vi "Convert register values.vi"(10 "Register strings":string[](array[string]), 11 "Register clusters":T1[](array[typedef])) -> (2 "Register clusters out":T1[](array[typedef]), 3 "Register strings out":string[](array[string]))   [LabVIEW 2020, in "PIC-Device.lvclass"]
uses:
  PIC-Device.lvclass
  Controls/Register to Write.ctl
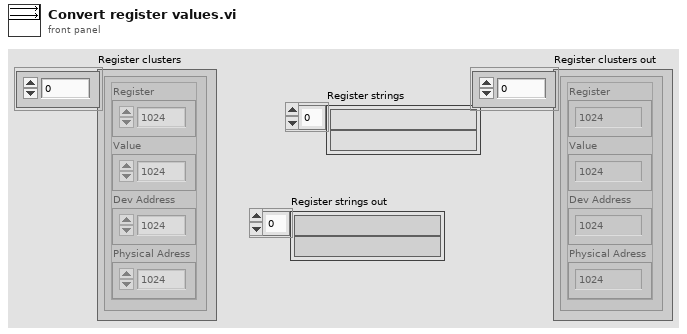
[diagram p1: front panel]
types:
  T1 = typedef "PIC-Device.lvclass/Register to Write.ctl" = cluster{"Register":u32, "Value":u32, "Dev Address":u32, "Physical Adress":u32}
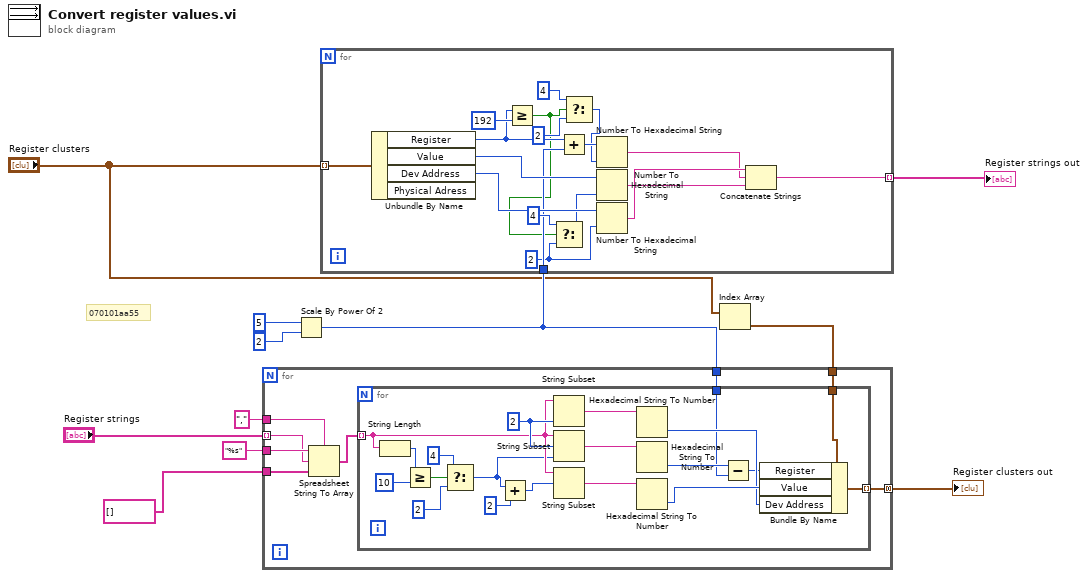
[diagram p0: block diagram]
diagram:
  # "070101aa55"
  n1 = Scale By Power Of 2(n=u32 5, x=u32 2) -> (x*2^n=w9:u32)
  n2 = for {
    tunnel: [w24] -> w7 mode=indexing
    tunnel: "Register clusters" -> [w23] mode=indexing
    tunnel: w9 -> [w15]
    w13 = i16 2 ("width (-)")
    n3 = Unbundle By Name(w23) -> ("Register"=w20:u32, "Value"=w22:u32, "Dev Address"=w28:u32)  [unwired: 1 out]
    n4 = Greater Or Equal?(x=w20, y=u32 192) -> (x >= y?=w12:bool)
    n5 = Select(t=i16 4 ("width (-)"), s=w12, f=w13) -> (s? t:f=w14:i16)
    n6 = Add(x=w20, y=w15) -> (x+y=w29:u32)
    n7 = Select(t=i16 4 ("width (-)"), s=w12, f=i16 2 ("width (-)")) -> (s? t:f=w17:i16)
    n8 = Number To Hexadecimal String(1:w17, 2:w29) -> (0:w26:string)
    n9 = Number To Hexadecimal String(1:w14, 2:w22) -> (0:w25:string)
    n10 = Number To Hexadecimal String(1:w13, 2:w28) -> (0:w27:string)
    n11 = Concatenate Strings(w27, w26, w25) -> (w24:string)
  }
  "Register strings out" <- w7
  n12 = Index Array(array="Register clusters") -> (element=w4:T1)  [unwired: 1 in]
  n13 = for {
    tunnel: "Register strings" -> [w31] mode=indexing
    tunnel: w9 -> [w35]
    tunnel: w4 -> [w37]
    tunnel: [w36] -> w6 mode=concatenating
    tunnel: string[] [] -> [w34]
    tunnel: "%s" ("format string") -> [w33]
    tunnel: "," ("delimiter (Tab)") -> [w32]
    n14 = Spreadsheet String To Array(delimiter (Tab)=w32, format string=w33, spreadsheet string=w31, array type (2D Dbl)=w34) -> (array=w30:string[])
    n15 = for {
      tunnel: w35 -> [w48]
      tunnel: w30 -> [w46] mode=indexing
      tunnel: w37 -> [w53]
      tunnel: [w52] -> w36 mode=indexing
      w57 = 2 ("length (rest)")
      n16 = String Length(string=w46) -> (length=w45:i32)
      n17 = Greater Or Equal?(x=w45, y=10) -> (x >= y?=w43:bool)
      n18 = Select(t=4 ("y"), s=w43, f=2 ("y")) -> (s? t:f=w40:i32)
      n19 = Add(x=w40, y=2 ("offset (0)")) -> (x+y=w38:i32)
      n20 = String Subset(string=w46, length (rest)=w57) -> (substring=w54:string)  [unwired: 1 in]
      n21 = String Subset(string=w46, offset (0)=w57, length (rest)=w40) -> (substring=w55:string)
      n22 = String Subset(string=w46, offset (0)=w38) -> (substring=w56:string)  [unwired: 1 in]
      n23 = Hexadecimal String To Number(string=w54) -> (number=w50:u32)  [unwired: 2 in, 1 out]
      n24 = Hexadecimal String To Number(string=w55) -> (number=w49:u32)  [unwired: 2 in, 1 out]
      n25 = Hexadecimal String To Number(string=w56) -> (number=w51:u32)  [unwired: 2 in, 1 out]
      n26 = Subtract(x=w49, y=w48) -> (x-y=w47:u32)
      n27 = Bundle By Name(cluster=w53, "Register"=w47, "Value"=w51, "Dev Address"=w50) -> (w52:T1)
    }
  }
  "Register clusters out" <- w6
